vi "RecordingDisplayCalculations_171213.vi"(10 "i":i32, 11 "DeCOutput":sgl[][](array[numeric])) -> (1 "Rel Y":sgl, 2 "Rel X":sgl, 3 "Mouse angle":sgl)   [LabVIEW 2016]
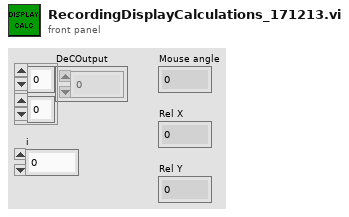
[diagram p1: front panel]
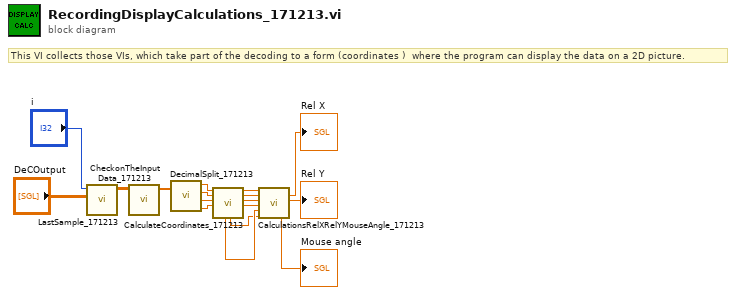
[diagram p0: block diagram]
diagram:
  # "This VI collects those VIs, which take part of the decoding to a form (coordinates )  where the program can display the data on a 2D picture."
  n1 = call "LastSample_171213.vi"("InputArray"="DeCOutput", "i"="i") -> ("OutputArray"=w7:sgl[][])  [unwired: 9 in]
  n2 = call "CheckonTheInputData_171213.vi"("InputArray"=w7) -> ("OutputArray"=w13:sgl[])  [unwired: 10 in]
  n3 = call "DecimalSplit_171213.vi"("InputArray"=w13) -> ("X1"=w14:sgl, "Y1"=w15:sgl, "X2"=w16:sgl, "Y2"=w17:sgl)  [unwired: 3 in]
  n4 = call "CalculateCoordinates_171213.vi"("X1"=w14, "Y1"=w15, "X2"=w16, "Y2"=w17) -> ("x1-x2"=w3:sgl, "y1-y2"=w2:sgl, "sina"=w6:sgl, "R from center"=w1:sgl, "Mouse Xc"=w5:sgl, "Mouse Yc"=w4:sgl)  [unwired: 8 in, 2 out]
  n5 = call "CalculationsRelXRelYMouseAngle_171213.vi"("sina"=w6, "R from center"=w1, "MouseXc"=w5, "Mouse Yc"=w4, "x1-x2"=w3, "y1-y2"=w2) -> ("Mouse angle"=→"Mouse angle":sgl, "Rel X"=→"Rel X":sgl, "Rel Y"=→"Rel Y":sgl)  [unwired: 7 in, 4 out]
